vi "SQL_Command.vi"(6 "Column":string[](array[string]), 11 "Table":string) -> (3 "SQL query":string)   [LabVIEW 2019]
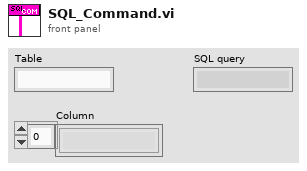
[diagram p1: front panel]
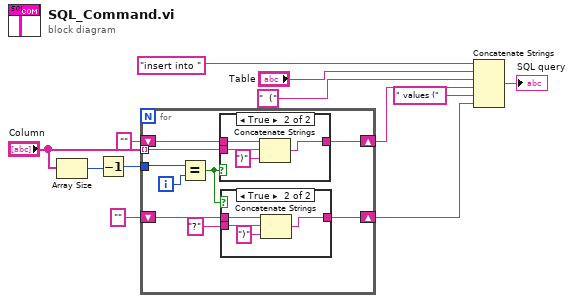
[diagram p0: block diagram]
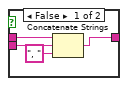
[diagram p2: hidden frame]
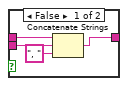
[diagram p3: hidden frame]
diagram:
  n1 = Array Size(array="Column") -> (size(s)=w5:i32)
  n2 = Decrement(x=w5) -> (x-1=w6:i32)
  n3 = for {
    tunnel: "Column" -> [w21] mode=indexing
    shift-right: [w20] -> w7
    shift-left: "" -> [w19]
    tunnel: w6 -> [w17]
    shift-right: [w16] -> w11
    shift-left: "" -> [w15]
    i -> [w18]
    n4 = Equal?(x=w17, y=w18) -> (x = y?=w13:bool)
    n5 = case shown="True" w13 {
      tunnel: w21 -> [w33 w35]
      tunnel: [w32 w36] -> w20
      tunnel: w19 -> [w31 w37]
      frame False {
        n6 = Concatenate Strings(w31, w33, ", " ("string")) -> (w32:string)
      }
      frame True {
        n7 = Concatenate Strings(w37, w35, ")" ("string")) -> (w36:string)
      }
    }
    n8 = case shown="True" w13 {
      tunnel: "?" -> [w25 w27]
      tunnel: [w24 w28] -> w16
      tunnel: w15 -> [w23 w29]
      frame False {
        n9 = Concatenate Strings(w23, w25, ", " ("string")) -> (w24:string)
      }
      frame True {
        n10 = Concatenate Strings(w29, w27, ")" ("string")) -> (w28:string)
      }
    }
  }
  n11 = Concatenate Strings("insert into ", "Table", "  (" ("string"), w7, " values (" ("string"), w11) -> (→"SQL query":string)
